vi "2HP_Convert serial string to Eng vals.vi"(0 "Serial buffer string (excluding FrameChar)":string) -> (3 "Pressures":sgl[][](graph), 4 "Atmospheric pressure (mbar)":sgl, 6 "External thermistor temperature (deg C)":sgl, 8 "Env. sensor die temperature (deg C)":sgl, 10 "Relative humidity (%)":sgl, 13 "All vals":sgl[](array[numeric]), 14 "Gyration vector (deg / s)":sgl[](array[numeric]), 15 "Acceleration vector (g)":sgl[](array[numeric]))   [LabVIEW 2020]
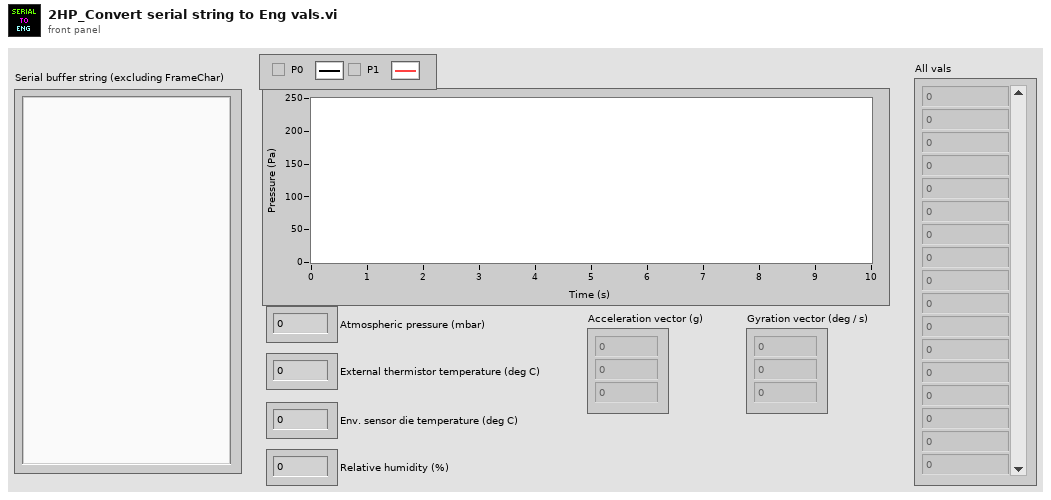
[diagram p1: front panel]
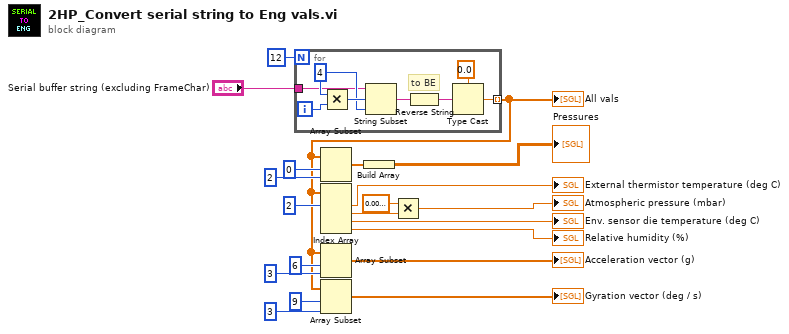
[diagram p0: block diagram]
diagram:
  n1 = for {
    N: 12 -> [_]
    tunnel: [w22] -> w6 mode=indexing
    tunnel: "Serial buffer string (excluding FrameChar)" -> [w21]
    i -> [w28]
    w26 = 4 ("x")
    # "to BE"
    n2 = Multiply(x=w26, y=w28) -> (x*y=w27:i32)
    n3 = String Subset(string=w21, offset (0)=w27, length (rest)=w26) -> (substring=w25:string)
    n4 = Reverse String(1:w25) -> (0:w24:string)
    n5 = Type Cast(type=sgl 0.0 ("byte count"), x=w24) -> (*(type *) &x=w22:sgl)
  }
  "All vals" <- w6
  n6 = Array Subset(array=w6, index=0, length=2) -> (w16:sgl[])
  n7 = Index Array(array=w6, index #1=2 ("index")) -> (element #1=→"External thermistor temperature (deg C)":sgl, element #2=w2:sgl, element #3=→"Env. sensor die temperature (deg C)":sgl, element #4=→"Relative humidity (%)":sgl)  [unwired: 3 in]
  n8 = Array Subset(array=w6, index=6, length=3) -> (→"Acceleration vector (g)":sgl[])
  n9 = Array Subset(array=w6, index=9, length=3) -> (→"Gyration vector (deg / s)":sgl[])
  n10 = Build Array(w16) -> (→"Pressures":sgl[][])
  n11 = Multiply(x=sgl 0.01, y=w2) -> (x*y=→"Atmospheric pressure (mbar)":sgl)
